vi "AddDataArryLimit.vi"(0 "MainDataArryIn":dbl[][](array[numeric]), 1 "SubDataArry":dbl[][](array[numeric]), 3 "MaxLength":i32=70000) -> (14 "输出数组":dbl[][](array[numeric]))   [LabVIEW 2020]
panel:
  # "MainDataArryOut"
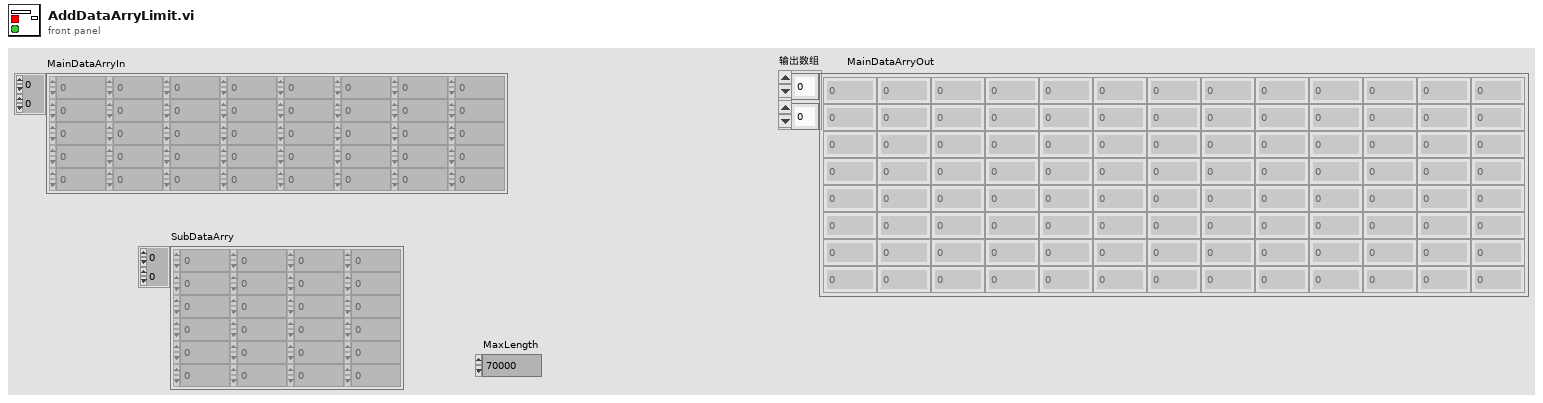
[diagram p1: front panel]
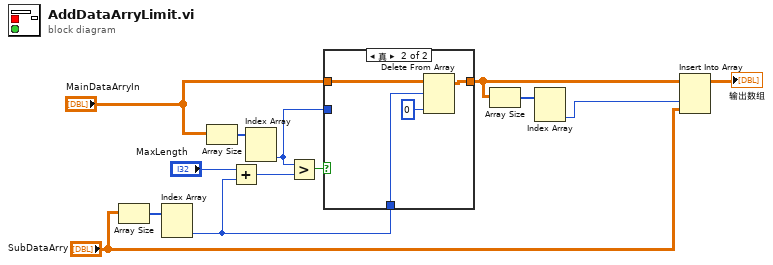
[diagram p0: block diagram]
diagram:
  n1 = Array Size(array="SubDataArry") -> (size(s)=w4:i32[])
  n2 = Index Array(array=w4) -> (element #2=w3:i32)  [unwired: 2 in, 1 out]
  n3 = Array Size(array="MainDataArryIn") -> (size(s)=w11:i32[])
  n4 = Add(x="MaxLength", y=w3) -> (x+y=w1:i32)
  n5 = Index Array(array=w11) -> (element #2=w8:i32)  [unwired: 2 in, 1 out]
  n6 = Greater?(x=w8, y=w1) -> (0:w10:bool)
  n7 = case shown="真" w10 {
    tunnel: "MainDataArryIn" -> [w14 w18]
    tunnel: [w14 w17] -> w9
    tunnel: w8 -> [_ _]
    tunnel: w3 -> [_ w15]
    frame False {
    }
    frame True {
      n8 = Delete From Array(array=w18, length=w15, index (col)=0 ("禁用的索引 (列)")) -> (array with subset deleted=w17:dbl[][])  [unwired: 1 in, 1 out]
    }
  }
  n9 = Array Size(array=w9) -> (size(s)=w13:i32[])
  n10 = Index Array(array=w13) -> (element #2=w12:i32)  [unwired: 2 in, 1 out]
  n11 = Insert Into Array(array=w9, index (col)=w12, new element="SubDataArry") -> (→"输出数组":dbl[][])  [unwired: 1 in]
